vi "Multiply Amplitude by Output Gain.vi"(8 "error in (no error)":errorcluster, 11 "Instrument.DAQ":refnum<class "Instrument.DAQ.lvclass">) -> (0 "error out":errorcluster, 3 "Instrument.DAQ out":refnum<class "Instrument.DAQ.lvclass">)   [LabVIEW 2019, in "Instrument.Lockin.lvlib" / "Instrument.DAQ.lvclass"]
uses:
  Instrument.DAQ.lvclass
  Typedefs/AO.Channel--Cluster--Array.ctl
  Typedefs/AO.Channel--Cluster.ctl
  Typedefs/AO.Channel.Function--Enum.ctl
panel:
  out "Cfg_AO":T1 {"Phase" format="%#_3g"; "Frequency" min=0.0001 max=200000.0 format="%#_6p"; "Offset" format="%#_6p"; "Amplitude" min=0.0 max=10.0 format="%#_6p"}
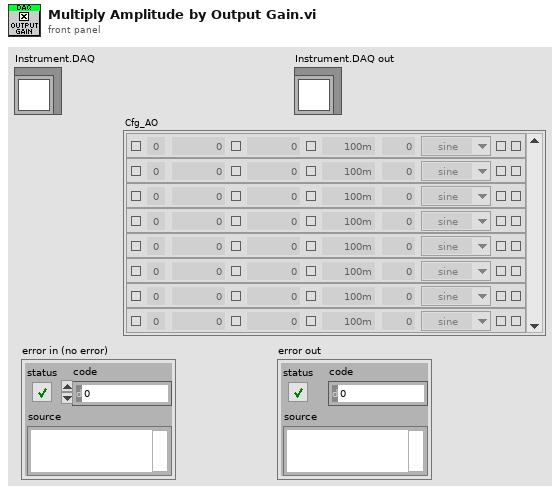
[diagram p1: front panel]
types:
  T1 = typedef "Instrument.Lockin.lvlib/Instrument.DAQ.lvclass/AO.Channel--Cluster--Array.ctl" = T2[]
  T2 = typedef "Instrument.Lockin.lvlib/Instrument.DAQ.lvclass/AO.Channel--Cluster.ctl" = cluster{"Enable?":bool, "Channel":i32, "Amplitude":dbl, "Offset":dbl, "Frequency":dbl, "Phase":dbl, "Function":T3, "Sweeping?":bool, "Limit AC":bool, "Limit DC?":bool, "Duty Cycle":bool}
  T3 = typedef "Instrument.Lockin.lvlib/Instrument.DAQ.lvclass/AO.Channel.Function--Enum.ctl" = enum16{"sine", "square", "triangle", "saw"}
  T4 = typedef "Instrument.Lockin.lvlib/Instrument.DAQ.lvclass/Channel.Gain--Cluster--Array.ctl" = T5[]
  T5 = typedef "Instrument.Lockin.lvlib/Instrument.DAQ.lvclass/Channel.Gain--Cluster.ctl" = cluster{"Channel":string, "Gain":dbl}
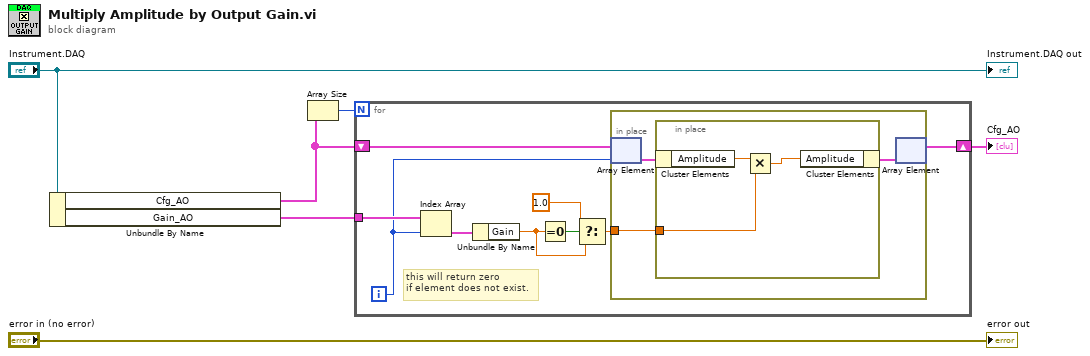
[diagram p0: block diagram]
diagram:
  n1 = Unbundle By Name("Instrument.DAQ") -> ("Cfg_AO"=w1:T1, "Gain_AO"=w3:T4)
  n2 = Array Size(array=w1) -> (size(s)=w4:i32)
  n3 = for {
    N: w4 -> [_]
    tunnel: w3 -> [w11]
    shift-right: [w15] -> w2
    shift-left: w1 -> [w14]
    i -> [w9]
    # "this will return zero\nif element does not exist."
    n4 = Index Array(array=w11, index=w9) -> (element=w8:T5)
    n5 = Unbundle By Name(w8) -> ("Gain"=w7:dbl)
    n6 = Equal To 0?(x=w7) -> (x = 0?=w13:bool)
    n7 = Select(t=1.0, s=w13, f=w7) -> (s? t:f=w10:dbl)
    n8 = in-place {
      in-place-border: w10 -> [w18]
      n9 = in-place-array #1(w14, w9) -> (w17:T2)
      n10 = in-place {
        in-place-border: w18 -> [w21]
        n11 = in-place-cluster #2(w17) -> ("Amplitude"=w20:dbl)
        n12 = Multiply(x=w20, y=w21) -> (x*y=w19:dbl)
        n13 = in-place-cluster #2("Amplitude"=w19) -> (w16:T2)
      }
      n14 = in-place-array #1(w16) -> (w15:T1)  [unwired: 1 out]
    }
  }
  "Cfg_AO" <- w2
  "error out" <- "error in (no error)"
  "Instrument.DAQ out" <- "Instrument.DAQ"
